vi "Normalize Coordinates A.vi"(6 "Score":dbl, 8 "Center":cluster{"X":dbl, "Y":dbl}, 9 "Distance":dbl, 10 "Bounding box":T3, 11 "Image in":T1) -> (1 "Results":T2 {"Score" format="%#_3g"; "Pixels"."Rectangle"."Numeric 5" format="%#_3g"; "Pixels"."Rectangle"."Numeric 3" format="%#_3g"; "Pixels"."Rectangle"."Numeric 2" format="%#_3g"; "Pixels"."Rectangle"."Numeric" format="%#_3g"; "Normalized"."Rectangle"."Numeric 5" format="%#_2g"; "Normalized"."Rectangle"."Numeric 3" format="%#_2g"; "Normalized"."Rectangle"."Numeric 2" format="%#_2g"; "Normalized"."Rectangle"."Numeric" format="%#_2g"; "Normalized"."Center"."?" format="%#_3g"; "Normalized"."Center"."?" format="%#_3g"; "Distance (ft)" format="%#_3g"}, 2 "Center":dbl format="%.6g", 3 "Image out":T1)   [LabVIEW 2025]
doc: "Normalize the rectangle and center so that they range from -1 to 1, left to right and bottom to top. This helps with producing joystick coordinates for driving the robot and makes the code better at handling resolution changes of the camera."
uses:
  <vilib>/vision/Image Controls.llb/IMAQ Image.ctl
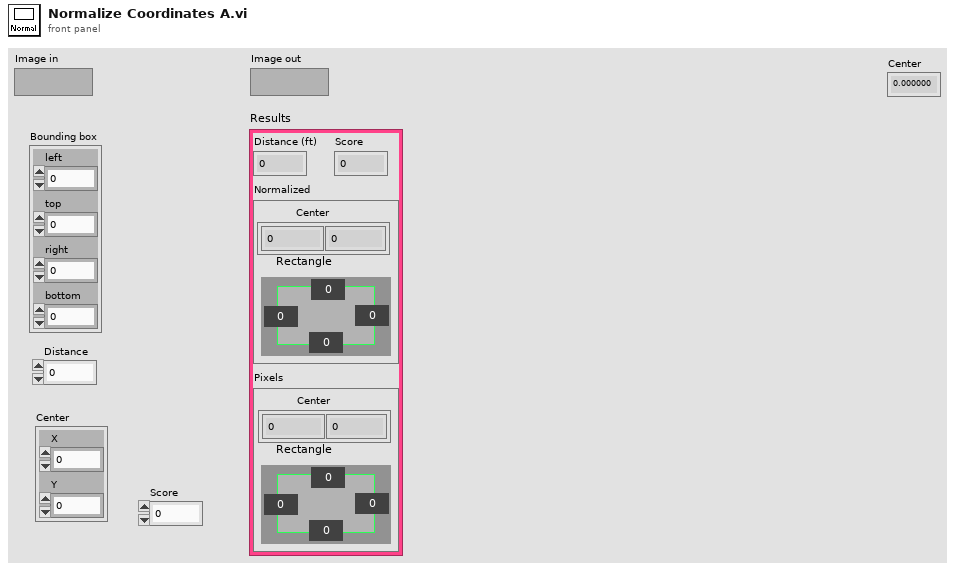
[diagram p1: front panel]
types:
  T1 = typedef "IMAQ Image.ctl" = refnum<image>
  T2 = cluster{"Distance (ft)":dbl, "Score":dbl, "Normalized":cluster{"Center":cluster{dbl, dbl}, "Rectangle":cluster{"Numeric":dbl, "Numeric 2":dbl, "Numeric 3":dbl, "Numeric 5":dbl}}, "Pixels":cluster{"Center":cluster{dbl, dbl}, "Rectangle":cluster{"Numeric":dbl, "Numeric 2":dbl, "Numeric 3":dbl, "Numeric 5":dbl}}}
  T3 = cluster{"left":dbl, "top":dbl, "right":dbl, "bottom":dbl}
  T4 = cluster{"X Resolution":i32, i32, "X Resolution":i32, i32}
  T5 = cluster{"Center":cluster{"X":dbl, "Y":dbl}, "Bounding box":cluster{"left":dbl, "top":dbl, "right":dbl, "bottom":dbl}}
  T6 = cluster{cluster{dbl, dbl}, cluster{dbl, dbl, dbl, dbl}}
  T7 = cluster{"Distance":dbl, "Score":dbl, cluster{cluster{dbl, dbl}, cluster{dbl, dbl, dbl, dbl}}, cluster{"Center":cluster{"X":dbl, "Y":dbl}, "Bounding box":cluster{"left":dbl, "top":dbl, "right":dbl, "bottom":dbl}}}
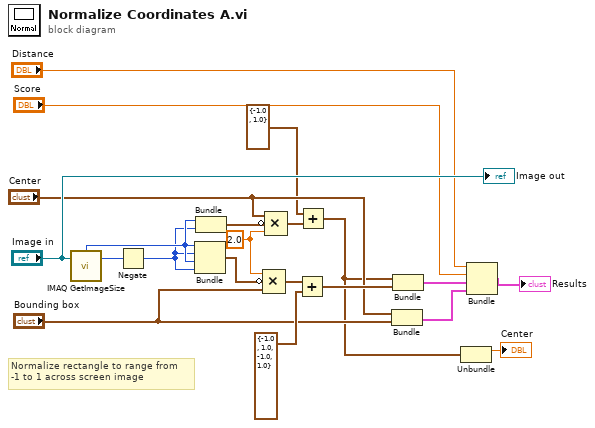
[diagram p0: block diagram]
diagram:
  w9 = 2.0
  # "Normalize rectangle to range from\n-1 to 1 across screen image"
  n1 = call "IMAQ GetImageSize"("Image"="Image in") -> ("Y Resolution"=w21:i32, "X Resolution"=w12:i32)  [unwired: 3 in, 1 out]
  n2 = Negate(x=w21) -> (-x=w11:i32)
  n3 = Bundle("X Resolution"=w12, w11, "X Resolution"=w12, w11) -> (w19:T4)  [unwired: 1 in]
  n4 = Bundle("X Resolution"=w12, w11) -> (w10:cluster{"X Resolution":i32, i32})  [unwired: 1 in]
  n5 = Compound Arithmetic op=MULTIPLY(w9, invert w19, "Bounding box") -> (w18:cluster{dbl, dbl, dbl, dbl})
  n6 = Compound Arithmetic op=MULTIPLY("Center", invert w10, w9) -> (w7:cluster{dbl, dbl})
  n7 = Add(x=w18, y=cluster{dbl, dbl, dbl, dbl} {-1.0, 1.0, -1.0, 1.0}) -> (x+y=w17:cluster{dbl, dbl, dbl, dbl})
  n8 = Add(x=cluster{dbl, dbl} {-1.0, 1.0} ("y"), y=w7) -> (x+y=w2:cluster{dbl, dbl})
  n9 = Bundle("Center"="Center", "Bounding box"="Bounding box") -> (w13:T5)  [unwired: 1 in]
  n10 = Bundle(w2, w17) -> (w3:T6)  [unwired: 1 in]
  n11 = Unbundle(w2) -> (→"Center":dbl)  [unwired: 1 out]
  n12 = Bundle("Distance"="Distance", "Score"="Score", w3, w13) -> (→"Results":T7)  [unwired: 1 in]
  "Image out" <- "Image in"
